vi "ToDB25Poow.vi"(11 "Power,%":dbl) -> (0 "cluster":T1)   [LabVIEW 2014]
panel:
  out "7":bool
  out "6":bool
  out "4":bool
  out "5":bool
  out "3":bool
  out "2":bool
  out "1":bool
  out "0":bool
  # "DB-25"
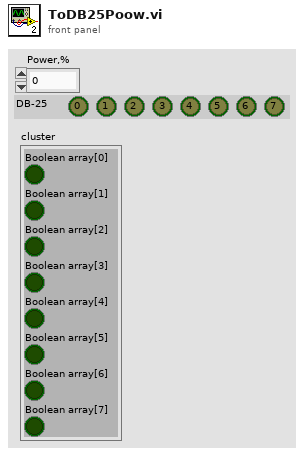
[diagram p1: front panel]
types:
  T1 = cluster{"Boolean array[0]":bool, "Boolean array[1]":bool, "Boolean array[2]":bool, "Boolean array[3]":bool, "Boolean array[4]":bool, "Boolean array[5]":bool, "Boolean array[6]":bool, "Boolean array[7]":bool}
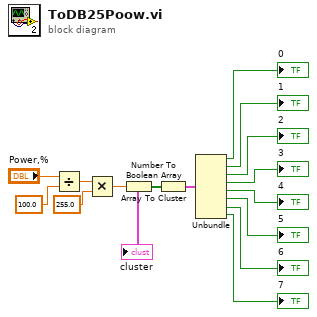
[diagram p0: block diagram]
diagram:
  n1 = Divide(x="Power,%", y=100.0) -> (x/y=w4:dbl)
  n2 = Multiply(x=w4, y=255.0) -> (x*y=w1:dbl)
  n3 = Number To Boolean Array(number=w1) -> (Boolean array=w15:bool[])
  n4 = Array To Cluster(array=w15) -> (cluster=w14:T1)
  "cluster" <- w14
  n5 = Unbundle(w14) -> ("Boolean array[0]"=→"0":bool, "Boolean array[1]"=→"1":bool, "Boolean array[2]"=→"2":bool, "Boolean array[3]"=→"3":bool, "Boolean array[4]"=→"4":bool, "Boolean array[5]"=→"5":bool, "Boolean array[6]"=→"6":bool, "Boolean array[7]"=→"7":bool)
